vi "Actor Core.vi"(8 "error in":errorcluster, 11 "TRExperimentsRaw in":refnum<class "Users.lvclass">) -> (0 "error out":errorcluster, 3 "Actor out":refnum<class "Actor.lvclass">)   [LabVIEW 2020, in "Forms.lvlib" / "Users.lvclass"]
doc: "The user interface for this panel.\n\n----\nPlease see the following web address for additional documentation and tutorial information:\nhttp://www.mooregoodideas.com/mgi-panel-manager/\n\nAuthor: Derek Trepanier\n\nCopyright (c) 2018, Moore Good Ideas, Inc.\n\nAll rights reserved.\n\nRedistribution and use in source and binary forms, with or without modification, are permitted provided that the following conditions are met:\n\n * Redistributions of source code must retain the above copyright notice, this list of conditions and the following disclaimer.\n * Redistributions in binary form must reproduce the above copyright notice, this list of conditions and the following disclaimer in the documentation and/or other materials provided with the distribution.\n * Neither the name of Moore Good Ideas, Inc. nor the names of its contributors may be used to endorse or promote products derived from this software without specific prior written permission.\n\nTHIS SOFTWARE IS PROVIDED BY THE COPYRIGHT HOLDERS AND CONTRIBUTORS \"AS IS\" AND ANY EXPRESS OR IMPLIED WARRANTIES, INCLUDING, BUT NOT LIMITED TO, THE IMPLIED WARRANTIES OF MERCHANTABILITY AND FITNESS FOR A PARTICULAR PURPOSE ARE DISCLAIMED. IN NO EVENT SHALL THE COPYRIGHT OWNER OR CONTRIBUTORS BE LIABLE FOR ANY DIRECT, INDIRECT, INCIDENTAL, SPECIAL, EXEMPLARY, OR CONSEQUENTIAL DAMAGES (INCLUDING, BUT NOT LIMITED TO, PROCUREMENT OF SUBSTITUTE GOODS OR SERVICES; LOSS OF USE, DATA, OR PROFITS; OR BUSINESS INTERRUPTION) HOWEVER CAUSED AND ON ANY THEORY OF LIABILITY, WHETHER IN CONTRACT, STRICT LIABILITY, OR TORT (INCLUDING NEGLIGENCE OR OTHERWISE) ARISING IN ANY WAY OUT OF THE USE OF THIS SOFTWARE, EVEN IF ADVISED OF THE POSSIBILITY OF SUCH DAMAGE."
uses:
  Users.lvclass
  C:/Users/User/Desktop/Raman Program/Database OOP/source/Forms AF/Form Controller/Panel Form Controller.lvclass
  <vilib>/ActorFramework/Actor/Actor.lvclass
  Forms Controller/Form Controller/Panel Form Controller.lvclass/Panel Form Controller.ctl
  Database OOP/Column Libraries/Basic Fields/Field Configurations/Field Configuration Class/Field Configuration.lvclass
  C:/Users/User/Desktop/Raman Program/Database OOP/source/Database OOP/Column Libraries/Field Interfaces/Field Configuration Interface Class/Field Configuration.lvclass
  Database OOP/Column Libraries/Basic Field Constructors/Text Field.vi
  Forms Controller/Form Window/Form Window.lvclass
  Database OOP/Table Libraries/Basic Form/Basic Form.lvclass
  Database OOP/Column Libraries/Basic Field Constructors.lvlib
  Forms Controller/Form Controller/Panel Form Controller.lvclass
panel:
  in  "Last Name":string
  in  "First Name":string
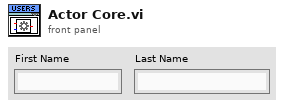
[diagram p1: front panel]
types:
  T1 = typedef "Panel Form Controller.lvlib/Builder Cluster.ctl" = cluster{"VI Ctrl Array":refnum<vi>[], "Form":refnum<class "Basic Form.lvclass">, "Open Form Button":refnum<class "Open Form Button.lvclass">}
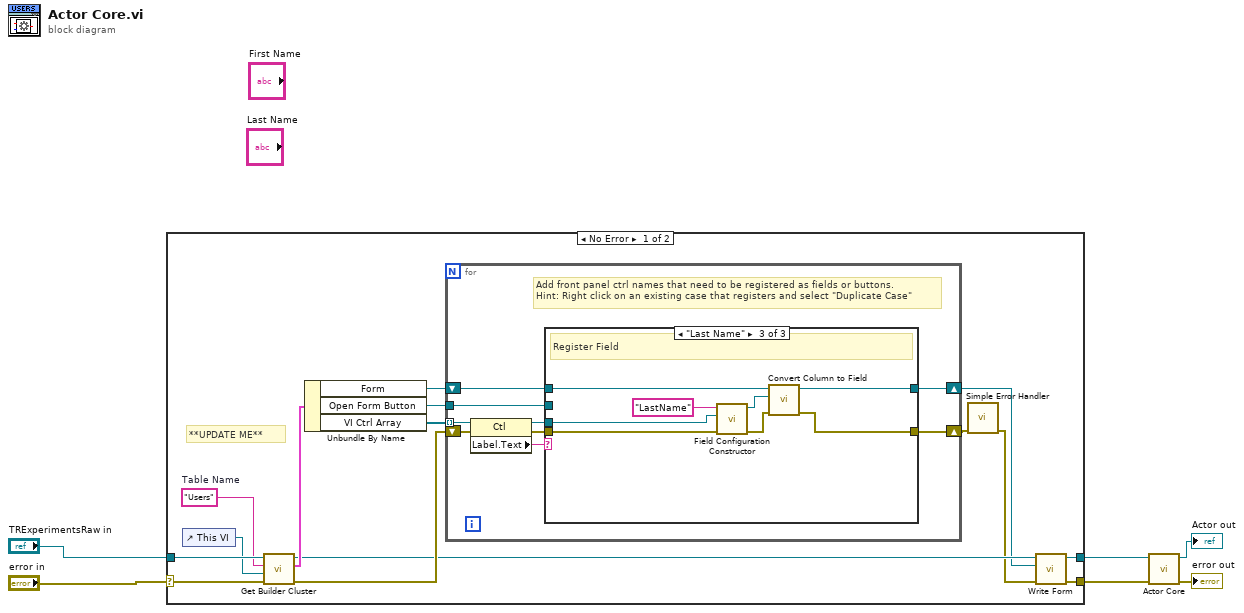
[diagram p0: block diagram]
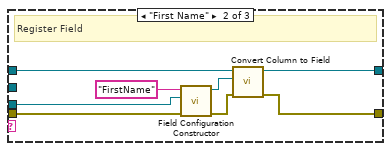
[diagram p3: hidden frame]
diagram:
  n1 = case shown="No Error" "error in" {
    selector: "error in" -> [w16 w50]
    tunnel: "TRExperimentsRaw in" -> [w20 w49]
    tunnel: [w9 w50] -> w2
    tunnel: [w10 w49] -> w1
    frame No Error {
      w7 = "Users"  # Table Name
      # "**UPDATE ME**"
      n2 = control-ref of="This VI"() -> (w8:refnum<vi>)
      n3 = call "Get Builder Cluster.vi"("error in (no error)"=w16, "VI Refnum"=w8, "Table Name"=w7, "Panel Form Controller in"=w20) -> ("error out"=w18:errorcluster, "Builder Cluster"=w17:T1, "Panel Form Controller out"=w13:refnum<class "Users.lvclass">)  [unwired: 5 in]
      n4 = Unbundle By Name(w17) -> ("Form"=w19:refnum<class "Basic Form.lvclass">, "Open Form Button"=w14:refnum<class "Open Form Button.lvclass">, "VI Ctrl Array"=w15:refnum<vi>[])
      n5 = for {
        tunnel: w15 -> [w30] mode=indexing
        shift-right: [w23] -> w11
        shift-left: w19 -> [w24]
        shift-right: [w28] -> w21
        shift-left: w18 -> [w27]
        tunnel: w14 -> [w22]
        # "Add front panel ctrl names that need to be registered as fields or buttons.\nHint: Right click on an existing case that registers and select \"Duplicate Case\""
        n6 = property class="Ctl"(reference=w30, error in=w27) -> (reference out=w29:refnum<vi>, error out=w26:errorcluster, "Label.Text"=w25:string)
        n7 = case shown="\"Last Name\"" w25 {
          tunnel: w29 -> [_ w35 w43]
          tunnel: w24 -> [w32 w40 w48]
          tunnel: [w32 w38 w46] -> w23
          tunnel: [w31 w39 w47] -> w28
          tunnel: w26 -> [w31 w34 w42]
          tunnel: w22 -> [_ _ _]
          frame "", Default {
            # "Not Registered"
          }
          frame "First Name" {
            # "Register Field"
            n8 = call-poly "Field Configuration Constructor.vi"("error in"=w34, "Ctl Refnum"=w35, "Column Name"="FirstName" ("Column")) -> ("error out"=w37:errorcluster, "Field Configuration"=w33:refnum<class "Field Configuration.lvclass">)  [unwired: 7 in]
            n9 = call "Convert Column to Field.vi"("error in (no error)"=w37, "Field Configuration"=w33, "Basic Form in"=w40) -> ("error out"=w39:errorcluster, "Basic Form out"=w38:refnum<class "Basic Form.lvclass">)  [unwired: 7 in]
          }
          frame "Last Name" {
            # "Register Field"
            n10 = call-poly "Field Configuration Constructor.vi"("error in"=w42, "Ctl Refnum"=w43, "Column Name"="LastName" ("Column")) -> ("error out"=w45:errorcluster, "Field Configuration"=w41:refnum<class "Field Configuration.lvclass">)  [unwired: 7 in]
            n11 = call "Convert Column to Field.vi"("error in (no error)"=w45, "Field Configuration"=w41, "Basic Form in"=w48) -> ("error out"=w47:errorcluster, "Basic Form out"=w46:refnum<class "Basic Form.lvclass">)  [unwired: 7 in]
          }
        }
      }
      n12 = call <vilib>:"Simple Error Handler.vi"("error in (no error)"=w21) -> ("error out"=w12:errorcluster)  [unwired: 4 in, 4 out]
      n13 = call "Write Form.vi"("error in (no error)"=w12, "Form.lvlib:Basic Form.lvclass"=w11, "Panel Form Controller in"=w13) -> ("error out"=w9:errorcluster, "Panel Form Controller out"=w10:refnum<class "Users.lvclass">)  [unwired: 7 in]
    }
    frame Error {
    }
  }
  n14 = call-parent "Actor Core.vi"("error in"=w2, "Form Window in"=w1) -> ("error out"=→"error out":errorcluster, "Actor out"=→"Actor out":refnum<class "Actor.lvclass">)  [unwired: 8 in]
